vi "Write error classifications.vi"(8 "error in":errorcluster, 10 "error classifications":T1[](array[typedef]), 11 "control module configuration in":refnum<class "control module configuration.lvclass">) -> (0 "error out":errorcluster, 3 "control module configuration out":refnum<class "control module configuration.lvclass">)   [LabVIEW 2013, in "control module configuration.lvclass"]
uses:
  control module configuration.lvclass
  error classification setting.ctl
  <vilib>/NI/Tag Bus Module Framework/runtime/error classification.ctl
  control module configuration.lvclass/control module configuration.ctl
  <vilib>/NI/Tag Bus Module Framework/runtime/TBM module execution interface.lvclass
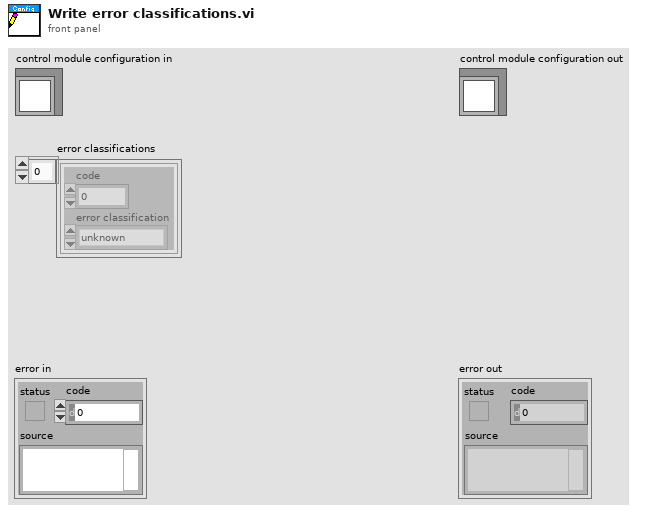
[diagram p1: front panel]
types:
  T1 = typedef "control module configuration.lvclass/error classification setting.ctl" = cluster{"code":i32, "error classification":T2}
  T2 = typedef "TBM module execution interface.lvclass/error classification.ctl" = enum16{"unknown", "none", "trivial", "recoverable", "critical"}
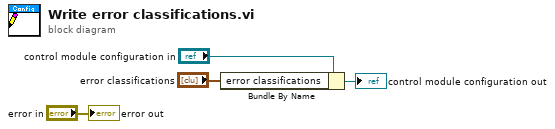
[diagram p0: block diagram]
diagram:
  n1 = Bundle By Name(cluster="control module configuration in", "error classifications"="error classifications") -> (→"control module configuration out":refnum<class "control module configuration.lvclass">)
  "error out" <- "error in"
